vi "WPILogInsertTimestampSortedRecord.vi"(9 "SizeIn":i32, 10 "Record":T1, 11 "Records":T1[](array[typedef])) -> (2 "SizeOut":i32, 3 "Array":T1[](array[typedef]))   [LabVIEW 2020]
uses:
  Typedef/Record.ctl
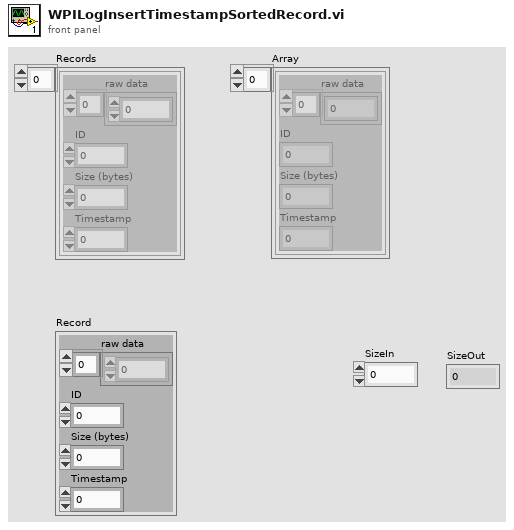
[diagram p1: front panel]
types:
  T1 = typedef "Record.ctl" = cluster{"raw data":u8[], "ID":u32, "Size (bytes)":u32, "Timestamp":u64}
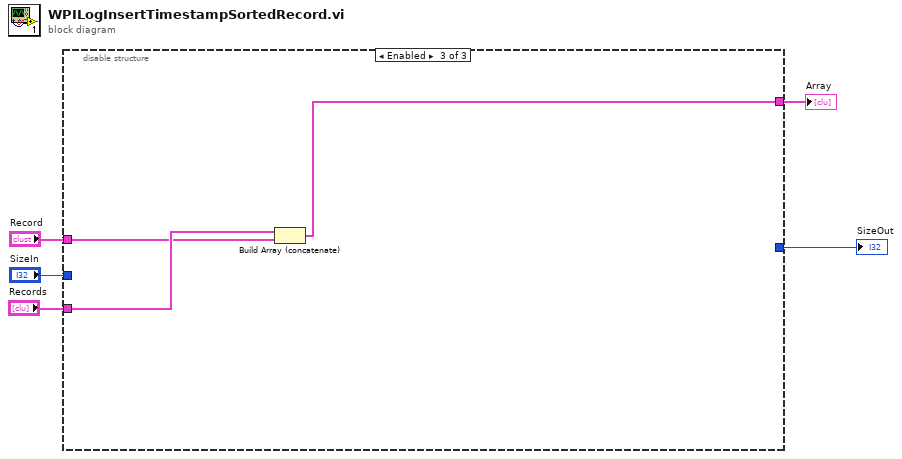
[diagram p0: block diagram]
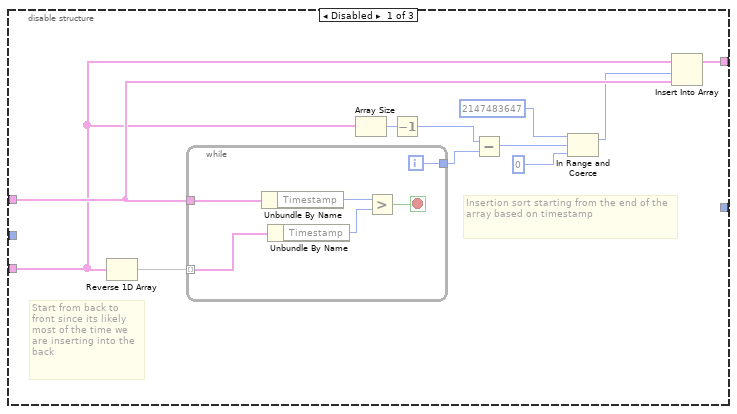
[diagram p2: hidden frame]
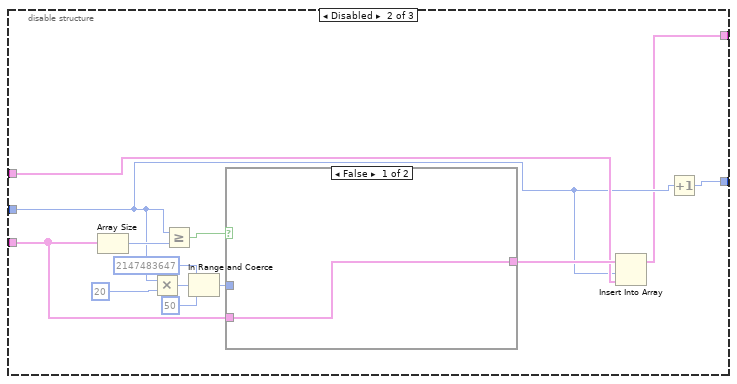
[diagram p3: hidden frame]
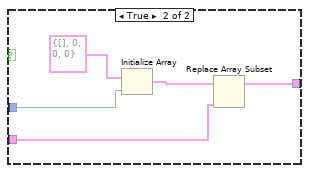
[diagram p4: hidden frame]
diagram:
  n1 = disable-structure shown="Enabled" {
    disable-tunnel: [w16 w23 w42] -> w5
    disable-tunnel: "Record" -> [w15 w25 w43]
    disable-tunnel: "Records" -> [w10 w31 w44]
    disable-tunnel: "SizeIn" -> [_ w24 _]
    disable-tunnel: [_ w30 _] -> w1
    frame Disabled {
      # "Insertion sort starting from the end of the array based on timestamp"
      # "Start from back to front since its likely most of the time we are inserting into the back"
      n2 = Reverse 1D Array(array=w10) -> (reversed array=w14:T1[])
      n3 = while {
        tunnel: w14 -> [w21] mode=indexing
        tunnel: w15 -> [w22]
        tunnel: [w17] -> w11
        i -> [w17]
        stop <- w18 stop-if-true
        n4 = Unbundle By Name(w22) -> ("Timestamp"=w20:u64)
        n5 = Unbundle By Name(w21) -> ("Timestamp"=w19:u64)
        n6 = Greater?(x=w20, y=w19) -> (0:w18:bool)
      }
      n7 = Array Size(array=w10) -> (size(s)=w13:i32)
      n8 = Decrement(x=w13) -> (x-1=w12:i32)
      n9 = Subtract(x=w12, y=w11) -> (x-y=w9:i32)
      n10 = In Range and Coerce(upper limit=2147483647, x=w9, lower limit=0) -> (coerced(x)=w7:i32)  [unwired: 1 out]
      n11 = Insert Into Array(array=w10, index=w7, new element=w15) -> (w16:T1[])
    }
    frame Disabled {
      n12 = Array Size(array=w31) -> (size(s)=w35:i32)
      n13 = Multiply(x=w24, y=20) -> (x*y=w33:i32)
      n14 = Greater Or Equal?(x=w24, y=w35) -> (x >= y?=w32:bool)
      n15 = In Range and Coerce(upper limit=2147483647, x=w33, lower limit=50) -> (coerced(x)=w28:i32)  [unwired: 1 out]
      n16 = case shown="False" w32 {
        tunnel: w28 -> [_ w41]
        tunnel: w31 -> [w36 w38]
        tunnel: [w36 w37] -> w29
        frame False {
        }
        frame True {
          n17 = Initialize Array(T1 {"raw data"=[], "ID"=0, "Size (bytes)"=0, "Timestamp"=0} ("Record"), w41) -> (w39:T1[])
          n18 = Replace Array Subset(array=w39, new element=w38) -> (w37:T1[])  [unwired: 1 in]
        }
      }
      n19 = Insert Into Array(array=w29, index=w24, new element=w25) -> (w23:T1[])
      n20 = Increment(x=w24) -> (x+1=w30:i32)
    }
    frame Enabled {
      n21 = Build Array (concatenate)(w44, w43) -> (w42:T1[])
    }
  }
  "Array" <- w5
  "SizeOut" <- w1
